vi "HV.vi"() -> ()   [LabVIEW 2015]
uses:
  GlobalPath.vi
  GlobalData.vi
  GlobalVi.vi
panel:
  in  "DONE WITH FINISHING?":bool
  in  "DONE WITH CABLING?":bool
  in  "DONE WITH GROUNDING?":bool
  in  "DONE WITH HV?":bool
  in  "ptfe 12":bool caption="Repeat for each PCB side: Conformal coating:\n1. Check the cleanliness of the HV filter region, if needed clean with alcohol and/or a metallic tip \n2. Carefully pour a small amount of conformal coating in a small cup\n3. Dip a brush into the liquid and carefully pass it over the HV filter components\n4. Visually check that the coating is uniformly applied and that the capacitor and resistance is covered\n5. Wait about 15 minutes for the coating to dry"
  in  "ptfe 7":bool caption="Repeat for each PCB side: Solder the HV cable (red) on the HV contact, where one lower end of the capacitor sits"
  in  "ptfe 11":bool caption="Repeat for each side of PCB1: Solder the grounding cable (black) on the grounding pad, where the 100 Ohm resistance sits"
  in  "ptfe 10":bool caption="Repeat for each panel corner: Electrically connect the cooling bar with the PCB ground:  \n1. Place the hole of the metallic eyelet on the cooling bar connnector hole\n2. Using a small screw, screw the eyelet on the cooling bar in such a way that the eyelet is facing towards the PCB ground\n3. Cut a piece of metallic cable, bend it in an L shape and solder it on one side on the eyelet and on the other on the PCB ground"
  in  "ptfe 6":bool caption="Repeat for each panel side: Solder the 100 Ohm grounding resistance between the PCB ground and the grounding pad"
  out "PanelName":string
  in  "ptfe 9":bool caption="Repeat for each panel junction: Using a metallic eyelet, electrically connect the adjacent PCB grounds"
  in  "DONE ALL ?":bool
  in  "ptfe 5":bool caption="Carefully clean the area with alcohol to get rid of soldering residuals"
  in  "ptfe 4":bool caption="Solder the resistance and capacitor"
  in  "ptfe 3":bool caption="Using thin tweezers position the 100 kOhm on top of the HV contact gap and \nthe 1 nF capacitor between the HV contact and the PCB ground"
  in  "ptfe 2":bool caption="Check that the HV contact region is clean and ready for soldering"
  # "1. HV filters (repeat for each PCB side)"
  # "2. Grounding"
  # "3. Cabling"
  # "4. Finishing"
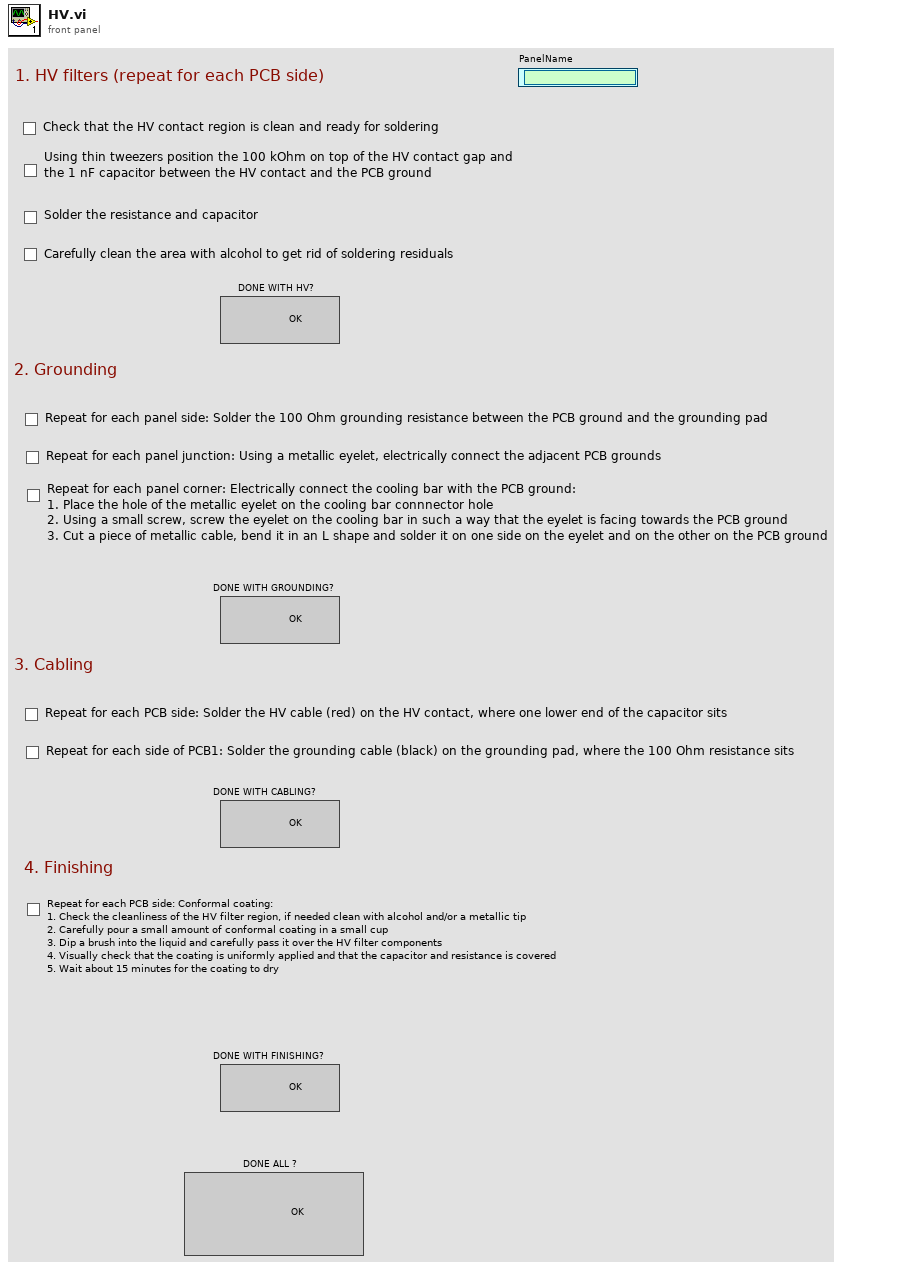
[diagram p1: front panel]
types:
  T1 = enum16{"open", "replace", "create", "open or create", "replace or create", "replace or create with confirmation"}
  T2 = enum32{"Bad", "Idle", "Run top level", "Running"}
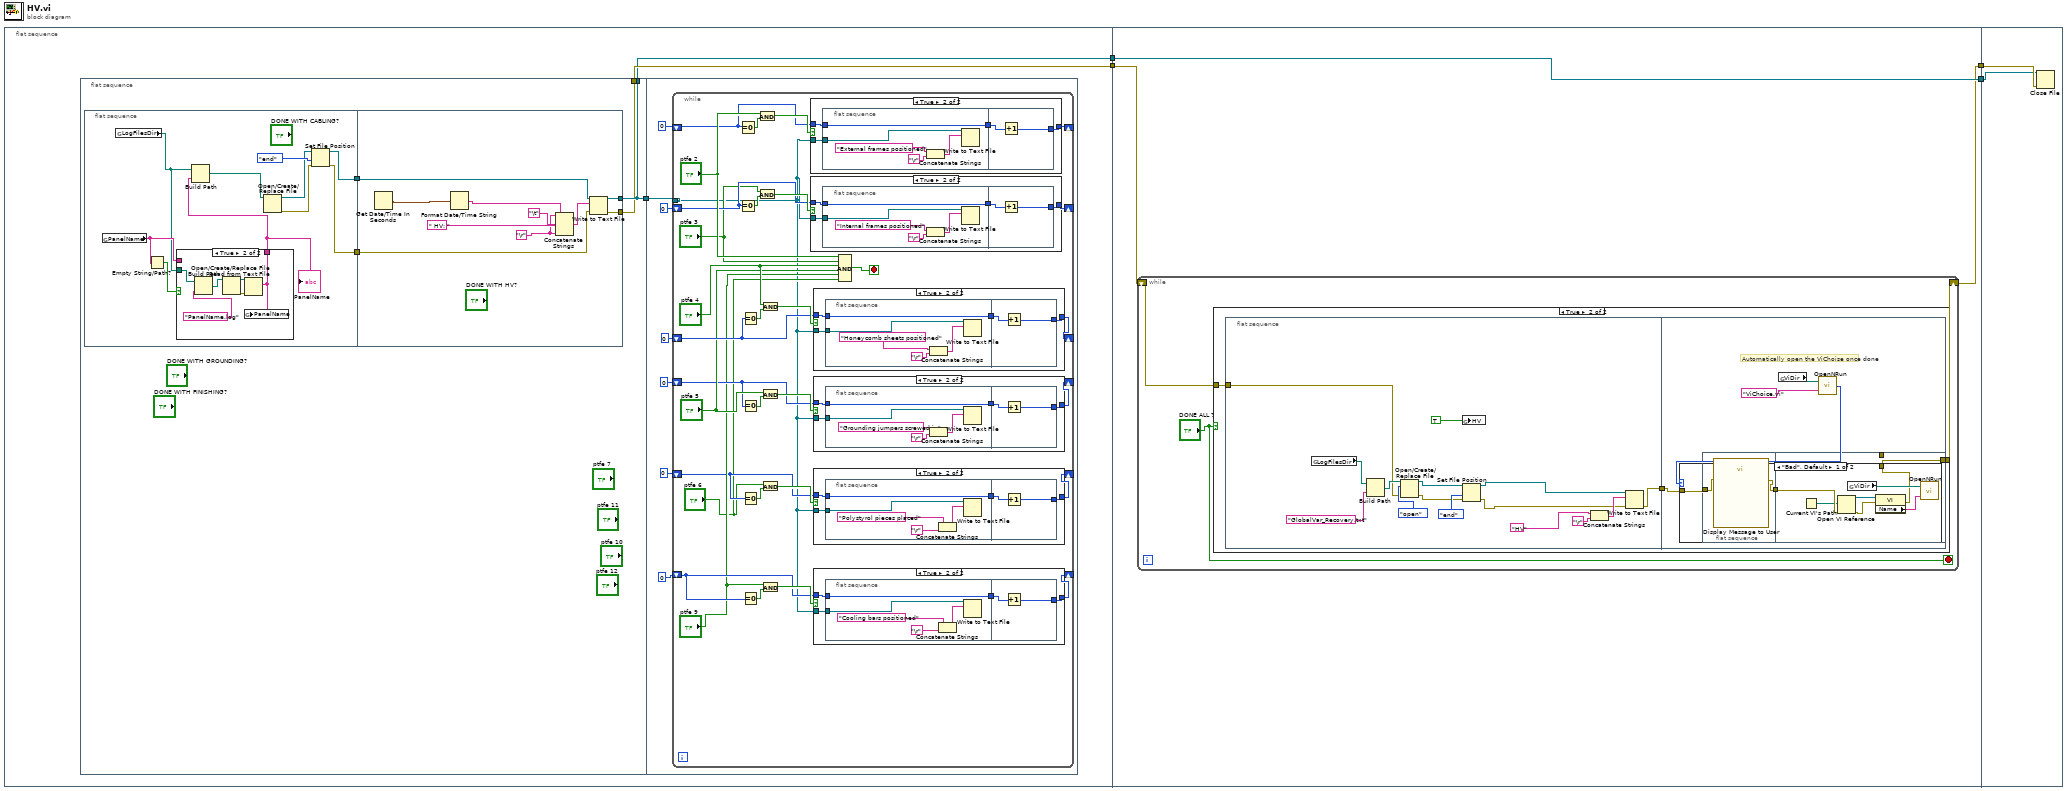
[diagram p0: block diagram]
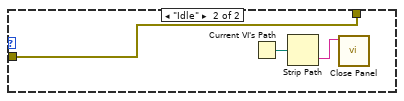
[diagram p10: hidden frame]
diagram:
  n1 = flat-sequence {
    tunnel: [w6] -> w3
    tunnel: [w5] -> w2
    tunnel: [w151] -> w4
    tunnel: w3 -> [w150]
    tunnel: w2 -> [w152]
    tunnel: [w152] -> w1
    tunnel: w4 -> [w196]
    tunnel: w1 -> [w195]
    frame #0 {
      n2 = flat-sequence {
        tunnel: [w10] -> w7
        tunnel: [w10] -> w5
        tunnel: [w9] -> w6
        tunnel: w7 -> [w45]
        frame #0 {
          n3 = flat-sequence {
            tunnel: [w16] -> w11
            tunnel: [w18] -> w8
            tunnel: w11 -> [w34]
            tunnel: [w33] -> w10
            tunnel: [w32] -> w9
            tunnel: w8 -> [w31]
            frame #0 {
              n4 = global read "GlobalData.vi" "PanelName"() -> (w15:string)
              n5 = global read "GlobalPath.vi" "LogFilesDir"() -> (w12:path)
              n6 = Empty String/Path?(string/path=w15) -> (empty?=w14:bool)
              n7 = case shown="True" w14 {
                tunnel: w12 -> [_ w28]
                tunnel: [w22 w23] -> w13
                tunnel: w15 -> [w22 _]
                frame False {
                }
                frame True {
                  n8 = Build Path(base path=w28, name or relative path="PanelName.log") -> (appended path=w27:path)
                  n9 = Open/Create/Replace File(file path (use dialog)=w27) -> (refnum out=w24:refnum<file>, error out=w25:errorcluster)  [unwired: 5 in, 1 out]
                  n10 = Read from Text File(file (use dialog)=w24, error in=w25) -> (text=w23:string)  [unwired: 2 in, 3 out]
                  n11 = global write "GlobalData.vi" "PanelName"(w23) -> ()
                }
              }
              "PanelName" <- w13
              n12 = Build Path(base path=w12, name or relative path=w13) -> (appended path=w21:path)
              n13 = Open/Create/Replace File(file path (use dialog)=w21) -> (refnum out=w17:refnum<file>, error out=w19:errorcluster)  [unwired: 5 in, 1 out]
              n14 = Set File Position(refnum=w17, from (0:start)=enum16{"start", "end", "current"}."end", error in=w19) -> (refnum out=w16:refnum<file>, error out=w18:errorcluster)  [unwired: 1 in]
            }
            frame #1 {
              w29 = "\r"
              n15 = Get Date/Time In Seconds() -> (seconds since 1Jan1904=w30:timestamp)
              n16 = Format Date/Time String(seconds (now)=w30) -> (date/time string=w36:string)  [unwired: 2 in]
              n17 = Concatenate Strings(w29, w36, "\t", " HV: ", w29) -> (w35:string)
              n18 = Write to Text File(file (use dialog)=w34, text=w35, error in=w31) -> (refnum out=w33:refnum<file>, error out=w32:errorcluster)  [unwired: 1 in, 1 out]
            }
          }
        }
        frame #1 {
          n19 = while {
            tunnel: w45 -> [w46]
            shift-right: [w72] -> _
            shift-left: 0 -> [w73]
            shift-right: [w68] -> _
            shift-left: 0 -> [w69]
            shift-right: [w62] -> _
            shift-left: 0 -> [w64]
            shift-right: [w57] -> _
            shift-left: 0 -> [w58]
            shift-right: [w53] -> _
            shift-left: 0 -> [w54]
            shift-right: [w48] -> _
            shift-left: 0 -> [w49]
            stop <- w77 stop-if-true
            n20 = Equal To 0?(x=w73) -> (x = 0?=w76:bool)
            n21 = Equal To 0?(x=w69) -> (x = 0?=w71:bool)
            n22 = Equal To 0?(x=w64) -> (x = 0?=w66:bool)
            n23 = Equal To 0?(x=w58) -> (x = 0?=w61:bool)
            n24 = Equal To 0?(x=w49) -> (x = 0?=w51:bool)
            n25 = Equal To 0?(x=w54) -> (x = 0?=w56:bool)
            n26 = And(x="ptfe 2", y=w76) -> (x .and. y?=w75:bool)
            n27 = And(x="ptfe 3", y=w71) -> (x .and. y?=w70:bool)
            n28 = And(x="ptfe 4", y=w66) -> (x .and. y?=w65:bool)
            n29 = And(x="ptfe 5", y=w61) -> (x .and. y?=w60:bool)
            n30 = And(x="ptfe 6", y=w51) -> (x .and. y?=w50:bool)
            n31 = And(x="ptfe 9", y=w56) -> (x .and. y?=w55:bool)
            n32 = case shown="True" w75 {
              tunnel: w46 -> [_ w142]
              tunnel: w73 -> [w138 w140]
              tunnel: [w138 w139] -> w72
              frame False {
              }
              frame True {
                n33 = flat-sequence {
                  tunnel: w142 -> [w145]
                  tunnel: [w144] -> w141
                  tunnel: w140 -> [w144]
                  tunnel: w141 -> [w149]
                  tunnel: [w148] -> w139
                  frame #0 {
                    n34 = Concatenate Strings("External frames positioned", "\r") -> (w147:string)
                    n35 = Write to Text File(file (use dialog)=w145, text=w147) -> ()  [unwired: 2 in, 3 out]
                  }
                  frame #1 {
                    n36 = Increment(x=w149) -> (x+1=w148:i32)
                  }
                }
              }
            }
            n37 = case shown="True" w70 {
              tunnel: w46 -> [_ w130]
              tunnel: w69 -> [w126 w128]
              tunnel: [w126 w127] -> w68
              frame False {
              }
              frame True {
                n38 = flat-sequence {
                  tunnel: w130 -> [w133]
                  tunnel: [w132] -> w129
                  tunnel: w128 -> [w132]
                  tunnel: w129 -> [w137]
                  tunnel: [w136] -> w127
                  frame #0 {
                    n39 = Concatenate Strings("Internal frames positioned", "\r") -> (w135:string)
                    n40 = Write to Text File(file (use dialog)=w133, text=w135) -> ()  [unwired: 2 in, 3 out]
                  }
                  frame #1 {
                    n41 = Increment(x=w137) -> (x+1=w136:i32)
                  }
                }
              }
            }
            n42 = case shown="True" w65 {
              tunnel: w46 -> [_ w118]
              tunnel: w64 -> [w114 w116]
              tunnel: [w114 w115] -> w62
              frame False {
              }
              frame True {
                n43 = flat-sequence {
                  tunnel: w118 -> [w121]
                  tunnel: [w120] -> w117
                  tunnel: w116 -> [w120]
                  tunnel: w117 -> [w125]
                  tunnel: [w124] -> w115
                  frame #0 {
                    n44 = Concatenate Strings("Honeycomb sheets positioned", "\r") -> (w123:string)
                    n45 = Write to Text File(file (use dialog)=w121, text=w123) -> ()  [unwired: 2 in, 3 out]
                  }
                  frame #1 {
                    n46 = Increment(x=w125) -> (x+1=w124:i32)
                  }
                }
              }
            }
            n47 = case shown="True" w60 {
              tunnel: w46 -> [_ w106]
              tunnel: w58 -> [w102 w104]
              tunnel: [w102 w103] -> w57
              frame False {
              }
              frame True {
                n48 = flat-sequence {
                  tunnel: w106 -> [w109]
                  tunnel: [w108] -> w105
                  tunnel: w104 -> [w108]
                  tunnel: w105 -> [w113]
                  tunnel: [w112] -> w103
                  frame #0 {
                    n49 = Concatenate Strings("Grounding jumpers screwed in", "\r") -> (w111:string)
                    n50 = Write to Text File(file (use dialog)=w109, text=w111) -> ()  [unwired: 2 in, 3 out]
                  }
                  frame #1 {
                    n51 = Increment(x=w113) -> (x+1=w112:i32)
                  }
                }
              }
            }
            n52 = case shown="True" w50 {
              tunnel: w46 -> [_ w82]
              tunnel: w49 -> [w78 w80]
              tunnel: [w78 w79] -> w48
              frame False {
              }
              frame True {
                n53 = flat-sequence {
                  tunnel: w82 -> [w85]
                  tunnel: [w84] -> w81
                  tunnel: w80 -> [w84]
                  tunnel: w81 -> [w89]
                  tunnel: [w88] -> w79
                  frame #0 {
                    n54 = Concatenate Strings("Polystyrol pieces placed", "\r") -> (w87:string)
                    n55 = Write to Text File(file (use dialog)=w85, text=w87) -> ()  [unwired: 2 in, 3 out]
                  }
                  frame #1 {
                    n56 = Increment(x=w89) -> (x+1=w88:i32)
                  }
                }
              }
            }
            n57 = case shown="True" w55 {
              tunnel: w46 -> [_ w94]
              tunnel: w54 -> [w90 w92]
              tunnel: [w90 w91] -> w53
              frame False {
              }
              frame True {
                n58 = flat-sequence {
                  tunnel: w94 -> [w97]
                  tunnel: [w96] -> w93
                  tunnel: w92 -> [w96]
                  tunnel: w93 -> [w101]
                  tunnel: [w100] -> w91
                  frame #0 {
                    n59 = Concatenate Strings("Cooling bars positioned", "\r") -> (w99:string)
                    n60 = Write to Text File(file (use dialog)=w97, text=w99) -> ()  [unwired: 2 in, 3 out]
                  }
                  frame #1 {
                    n61 = Increment(x=w101) -> (x+1=w100:i32)
                  }
                }
              }
            }
            n62 = Compound Arithmetic op=AND("ptfe 2", "ptfe 3", "ptfe 4", "ptfe 5", "ptfe 9", "ptfe 6") -> (w77:bool)
          }
        }
      }
    }
    frame #1 {
      n63 = while {
        shift-right: [w155] -> w151
        shift-left: w150 -> [w154]
        stop <- "DONE ALL ?" stop-if-true
        n64 = case shown="True" "DONE ALL ?" {
          tunnel: [w156 w159] -> w155
          tunnel: w154 -> [w156 w158]
          frame False {
          }
          frame True {
            n65 = flat-sequence {
              tunnel: w158 -> [w163]
              tunnel: [w162] -> w157
              tunnel: [w176] -> w159
              tunnel: w157 -> [w175]
              frame #0 {
                n66 = global read "GlobalPath.vi" "LogFilesDir"() -> (w160:path)
                n67 = Build Path(base path=w160, name or relative path="GlobalVar_Recovery.txt") -> (appended path=w172:path)
                n68 = Open/Create/Replace File(file path (use dialog)=w172, error in=w163, operation (0:open)=T1."open") -> (refnum out=w168:refnum<file>, error out=w169:errorcluster)  [unwired: 3 in, 1 out]
                n69 = global write "GlobalVi.vi" "HV"(TRUE) -> ()
                n70 = Set File Position(refnum=w168, from (0:start)=enum16{"start", "end", "current"}."end", error in=w169) -> (refnum out=w165:refnum<file>, error out=w164:errorcluster)  [unwired: 1 in]
                n71 = Concatenate Strings("HV", "\r") -> (w167:string)
                n72 = Write to Text File(file (use dialog)=w165, text=w167, error in=w164) -> (error out=w162:errorcluster)  [unwired: 1 in, 2 out]
              }
              frame #1 {
                # "Automatically open the ViChoise once done"
                n73 = global read "GlobalPath.vi" "ViDir"() -> (w179:path)
                n74 = call "OpenNRun.vi"("VI name"="ViChoice.vi", "ViDirPath"=w179) -> ("Execution:State"=w178:T2)
                n75 = case shown="\"Bad\", Default" w178 {
                  tunnel: [w180 w192] -> w176
                  tunnel: w175 -> [w181 w192]
                  frame "Bad", Default {
                    n76 = flat-sequence {
                      tunnel: w181 -> [w184]
                      tunnel: [w183] -> w182
                      tunnel: w182 -> [w188]
                      tunnel: [w185] -> w180
                      frame #0 {
                        n77 = call "Display Message to User"("error in (no error)"=w184) -> ("error out"=w183:errorcluster)  [unwired: 9 in, 1 out]
                      }
                      frame #1 {
                        n78 = Current VI's Path() -> (path=w186:path)
                        n79 = Open VI Reference(vi path=w186, error in (no error)=w188) -> (vi reference=w191:refnum<vi>, error out=w190:errorcluster)  [unwired: 4 in]
                        n80 = global read "GlobalPath.vi" "ViDir"() -> (w187:path)
                        n81 = property class="VI"(reference=w191, error in=w190) -> (error out=w185:errorcluster, "Name"=w189:string)  [unwired: 1 out]
                        n82 = call "OpenNRun.vi"("VI name"=w189, "ViDirPath"=w187) -> ()  [unwired: 1 out]
                      }
                    }
                  }
                  frame "Idle" {
                    n83 = Current VI's Path() -> (path=w193:path)
                    n84 = Strip Path(path=w193) -> (name=w194:string)  [unwired: 1 out]
                    n85 = call <vilib>:"Close Panel.vi"("VI name"=w194) -> ()  [unwired: 10 in, 1 out]
                  }
                }
              }
            }
          }
        }
      }
    }
    frame #2 {
      n86 = Close File(refnum=w195, error in=w196) -> ()  [unwired: 2 out]
    }
  }
